vi "RT Main.vi"   [LabVIEW 2016]
uses:
  <vilib>/FPGAPlugInAG/myRIO-1900/niLvFpga_Open_myRIO-1900.vi
  <vilib>/rvi/interface/common/dynamic/niFpgaDynamicAddResources.vi
  <vilib>/rvi/interface/nirviOpenFPGA/nirviOpenFPGA.xnode
  FPGA Bitfiles/MWefekty1_FPGATarget_FPGAMAIN_9O-mVqVYn1E.lvbitx
  FPGA_MAIN.vi
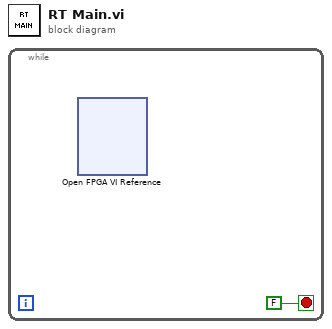
[diagram p0: block diagram]
diagram:
  n1 = while {
    stop <- FALSE stop-if-true
    n2 = xnode "Open FPGA VI Reference"() -> ()  [unwired: 2 in, 2 out]
  }
